vi "M227_Ctrl_Index.vi"(5 "OldVal":variant, 11 "NewVal":variant) -> (4 "Control Ref OUT":refnum<vi>, 8 "M227 Out":T1)   [LabVIEW 2014]
uses:
  Type Defs/M227.ctl
panel:
  in  "M227 In":T1
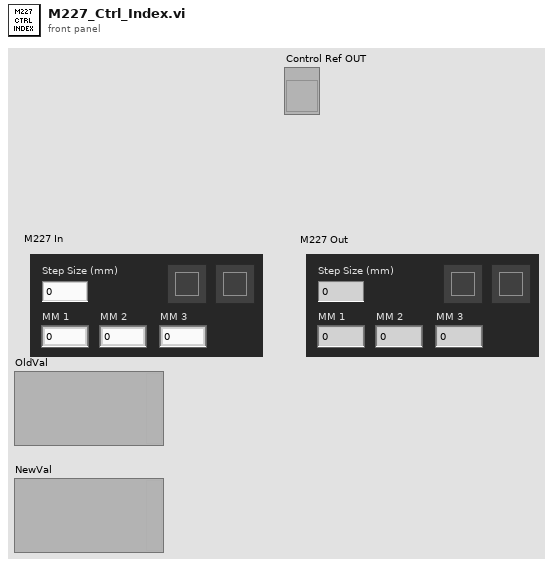
[diagram p1: front panel]
types:
  T1 = typedef "M227.ctl" = cluster{"Up M227":bool, "Down M227":bool, "Step Size (mm)":dbl, "MM 1":dbl, "MM 2":dbl, "MM 3":dbl}
  T2 = cluster{"Up M227":bool, "Down M227":bool, "Step Size (mm)":bool, "MM 1":bool, "MM 2":bool, "MM 3":bool}
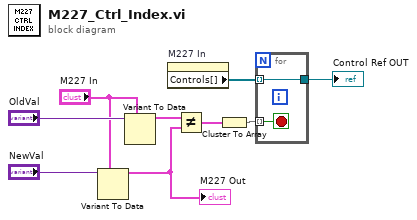
[diagram p0: block diagram]
diagram:
  n1 = Variant To Data(type="M227 In", Variant="NewVal") -> (data=w9:T1)  [unwired: 1 in, 1 out]
  "M227 Out" <- w9
  n2 = Variant To Data(type="M227 In", Variant="OldVal") -> (data=w4:T1)  [unwired: 1 in, 1 out]
  n3 = property on="M227 In" class="Clust"() -> ("Controls[]"=w1:refnum<vi>[])  [unwired: 2 in, 2 out]
  n4 = Not Equal?(x=w4, y=w9) -> (x != y?=w8:T2)
  n5 = Cluster To Array(cluster=w8) -> (array=w5:bool[])
  n6 = for {
    tunnel: w5 -> [w10] mode=indexing
    tunnel: w1 -> [w11] mode=indexing
    tunnel: [w11] -> w3
    stop <- w10 stop-if-true
  }
  "Control Ref OUT" <- w3
